vi "FP behavior FWD obstacle avoidance.vi"(1 "Behavior\nVelocity":dbl=20.0, 2 "Activate?":bool=TRUE, 3 "IR Sensors":T1(array[cluster])) -> (0 "Obs Avoid Array":dbl[](array[numeric]))   [LabVIEW 2014]
doc: "This vi uses the values from the Bow sensor to create an Obstacle Avoidance Array."
panel:
  out "Before Scaling":cluster{dbl, dbl, dbl[]}(graph)
  out "Waveform Graph":cluster{dbl, dbl, dbl[]}(graph)
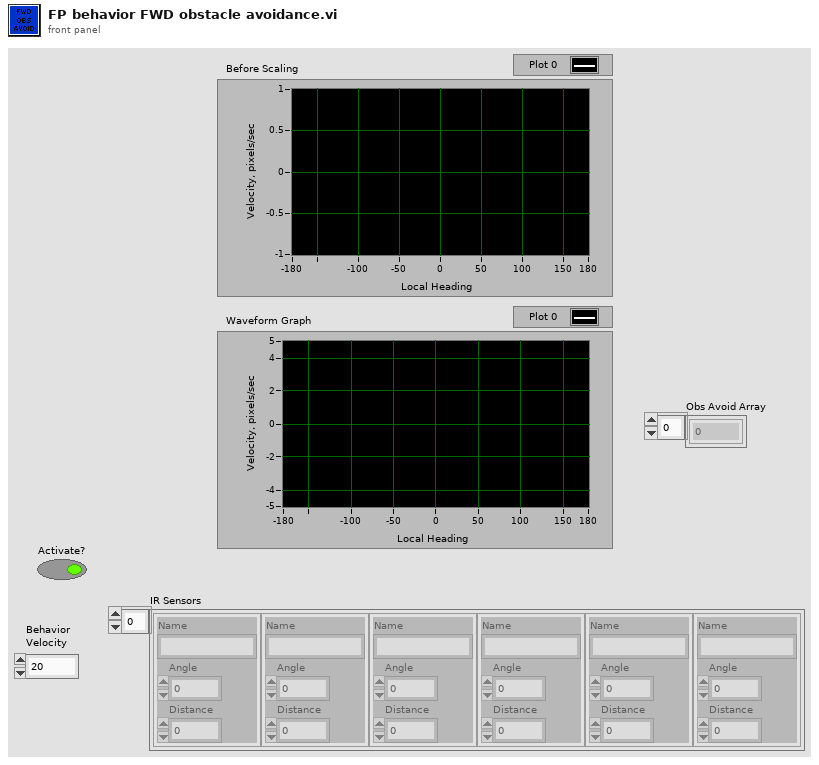
[diagram p1: front panel]
types:
  T1 = cluster{"Name":string, "Angle":dbl, "Distance":dbl}[]
  T2 = cluster{"Name":string, "Angle":dbl, "Distance":dbl}
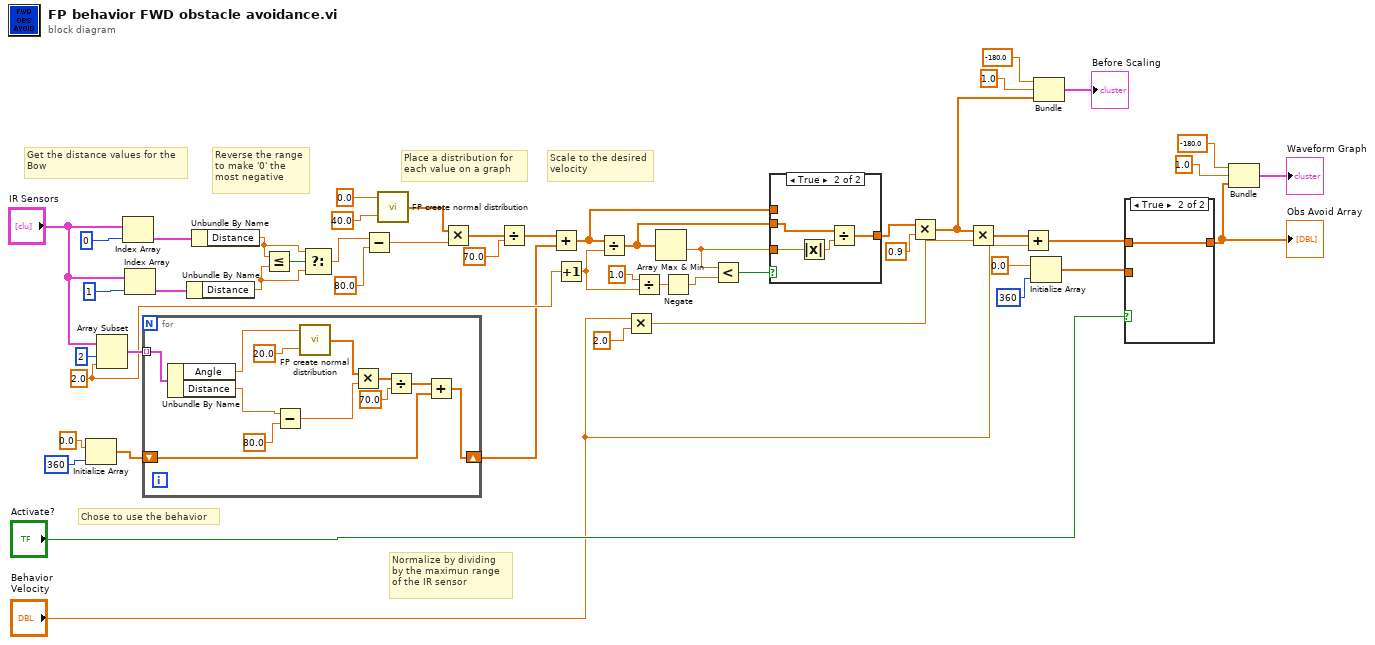
[diagram p0: block diagram]
diagram:
  w24 = 2.0 ("length")
  # "Scale to the desired\nvelocity"
  # "Chose to use the behavior"
  # "Reverse the range\nto make '0' the\nmost negative"
  # "Normalize by dividing\nby the maximun range\nof the IR sensor"
  # "Place a distribution for \neach value on a graph"
  # "Get the distance values for the\nBow"
  n1 = Initialize Array(0.0 ("element"), 360 ("dimension size")) -> (w25:dbl[])
  n2 = Array Subset(array="IR Sensors", index=2, length=w24) -> (w29:T1)
  n3 = Index Array(array="IR Sensors", index=0) -> (element=w50:T2)
  n4 = Index Array(array="IR Sensors", index=1) -> (element=w34:T2)
  n5 = for {
    tunnel: w29 -> [w63] mode=indexing
    shift-right: [w54] -> w15
    shift-left: w25 -> [w55]
    n6 = Unbundle By Name(w63) -> ("Angle"=w61:dbl, "Distance"=w53:dbl)
    n7 = Subtract(x=w53, y=80.0) -> (x-y=w60:dbl)
    n8 = call "FP create normal distribution.vi"("std (Normal)"=20.0, "mean"=w61) -> ("ACT array"=w59:dbl[])
    n9 = Multiply(x=w59, y=w60) -> (x*y=w58:dbl[])
    n10 = Divide(x=w58, y=70.0) -> (x/y=w56:dbl[])
    n11 = Add(x=w56, y=w55) -> (x+y=w54:dbl[])
  }
  n12 = Unbundle By Name(w34) -> ("Distance"=w23:dbl)
  n13 = Unbundle By Name(w50) -> ("Distance"=w32:dbl)
  n14 = Less Or Equal?(x=w32, y=w23) -> (x <= y?=w33:bool)
  n15 = Select(t=w32, s=w33, f=w23) -> (s? t:f=w17:dbl)
  n16 = Subtract(x=w17, y=80.0) -> (x-y=w44:dbl)
  n17 = call "FP create normal distribution.vi"("std (Normal)"=40.0, "mean"=0.0) -> ("ACT array"=w26:dbl[])
  n18 = Multiply(x=w26, y=w44) -> (x*y=w43:dbl[])
  n19 = Divide(x=w43, y=70.0) -> (x/y=w16:dbl[])
  n20 = Add(x=w16, y=w15) -> (x+y=w11:dbl[])
  n21 = Increment(x=w24) -> (x+1=w8:dbl)
  n22 = Divide(x=w11, y=w8) -> (x/y=w10:dbl[])
  n23 = Multiply(x="Behavior\nVelocity", y=2.0) -> (x*y=w37:dbl)
  n24 = Divide(x=1.0, y=w8) -> (x/y=w7:dbl)
  n25 = Array Max & Min(array=w10) -> (min value=w13:dbl)  [unwired: 3 out]
  n26 = Negate(x=w7) -> (-x=w6:dbl)
  n27 = Less?(x=w13, y=w6) -> (x < y?=w12:bool)
  n28 = case shown="True" w12 {
    tunnel: w11 -> [w64 _]
    tunnel: [w64 w68] -> w3
    tunnel: w13 -> [_ w66]
    tunnel: w10 -> [_ w65]
    frame False {
    }
    frame True {
      n29 = Absolute Value(x=w66) -> (abs(x)=w67:dbl)
      n30 = Divide(x=w65, y=w67) -> (x/y=w68:dbl[])
    }
  }
  n31 = Multiply(x=w3, y=0.9) -> (x*y=w4:dbl[])
  n32 = Multiply(x=w4, y=w37) -> (x*y=w21:dbl[])
  n33 = Add(x=w21, y="Behavior\nVelocity") -> (x+y=w1:dbl[])
  n34 = Initialize Array(0.0 ("element"), 360 ("dimension size")) -> (w5:dbl[])
  n35 = Bundle(-180.0, 1.0, w4) -> (→"Before Scaling":cluster{dbl, dbl, dbl[]})  [unwired: 1 in]
  n36 = case shown="True" "Activate?" {
    tunnel: w1 -> [_ w70]
    tunnel: w5 -> [w69 _]
    tunnel: [w69 w70] -> w39
    frame False {
    }
    frame True {
    }
  }
  "Obs Avoid Array" <- w39
  n37 = Bundle(-180.0, 1.0, w39) -> (→"Waveform Graph":cluster{dbl, dbl, dbl[]})  [unwired: 1 in]
